vi "Port Read (SubVI).vi"(0 "VISA Refnum in":refnum<visa-resource-name>, 1 "error in":errorcluster) -> (2 "VISA Refnum out":refnum<visa-resource-name>, 3 "chaîne concaténée":string, 4 "nombre":dbl, 5 "error out":errorcluster)   [LabVIEW 2017]
doc: "Read data from the VISA Refnum, read the full (as Bytes as the COM port is configured) message from the COM port.\nMade by Tanguy BOULARD\nTHALES FRANCE"
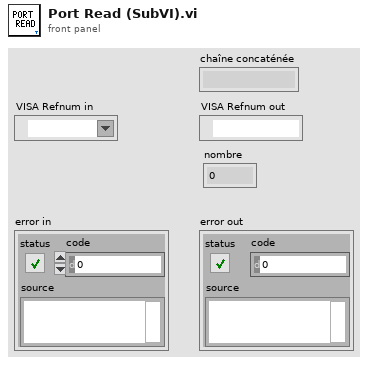
[diagram p1: front panel]
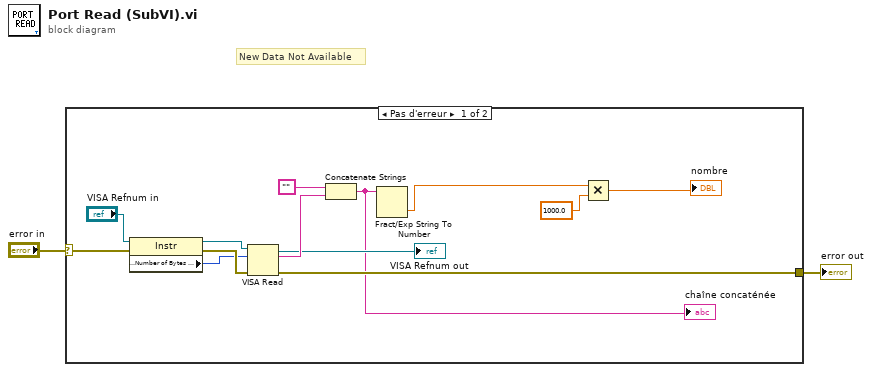
[diagram p0: block diagram]
diagram:
  # "New Data Not Available"
  n1 = case shown="Pas d'erreur" "error in" {
    selector: "error in" -> [w15 w16]
    tunnel: [w14 w16] -> w2
    frame No Error {
      n2 = property class="Instr"(reference="VISA Refnum in", error in=w15) -> (reference out=w10:refnum<visa-resource-name>, error out=w9:errorcluster, "Serial Settings:Number of Bytes at Serial Port"=w8:u32)
      n3 = VISA Read(VISA resource name=w10, byte count=w8, error in (no error)=w9) -> (VISA resource name out=→"VISA Refnum out":refnum<visa-resource-name>, read buffer=w12:string, error out=w14:errorcluster)  [unwired: 1 out]
      n4 = Concatenate Strings("", w12) -> (w6:string)
      "chaîne concaténée" <- w6
      n5 = Fract/Exp String To Number(string=w6) -> (number=w5:dbl)  [unwired: 3 in, 1 out]
      n6 = Multiply(x=w5, y=1000.0) -> (x*y=→"nombre":dbl)
    }
    frame Error {
    }
  }
  "error out" <- w2
